vi "Database.UpdateVariantFiles.vi"(8 "error in":errorcluster) -> (0 "error out":errorcluster)   [LabVIEW 2016]
uses:
  Global/ApplicationGlobal.vi
  Logger/Logger.FileBody.ctl
panel:
  out "HandledFileContent":T1[](array[typedef]) {"Values" format="%.3f"}
  out "HandledFileContent":T1 {"Values" format="%.3f"}
  out "Array":string[](array[string])
  out "text":string
  out "SerialNo":string
  out "Variant":string
  out "System":string
  out "filenames":string[](array[string])
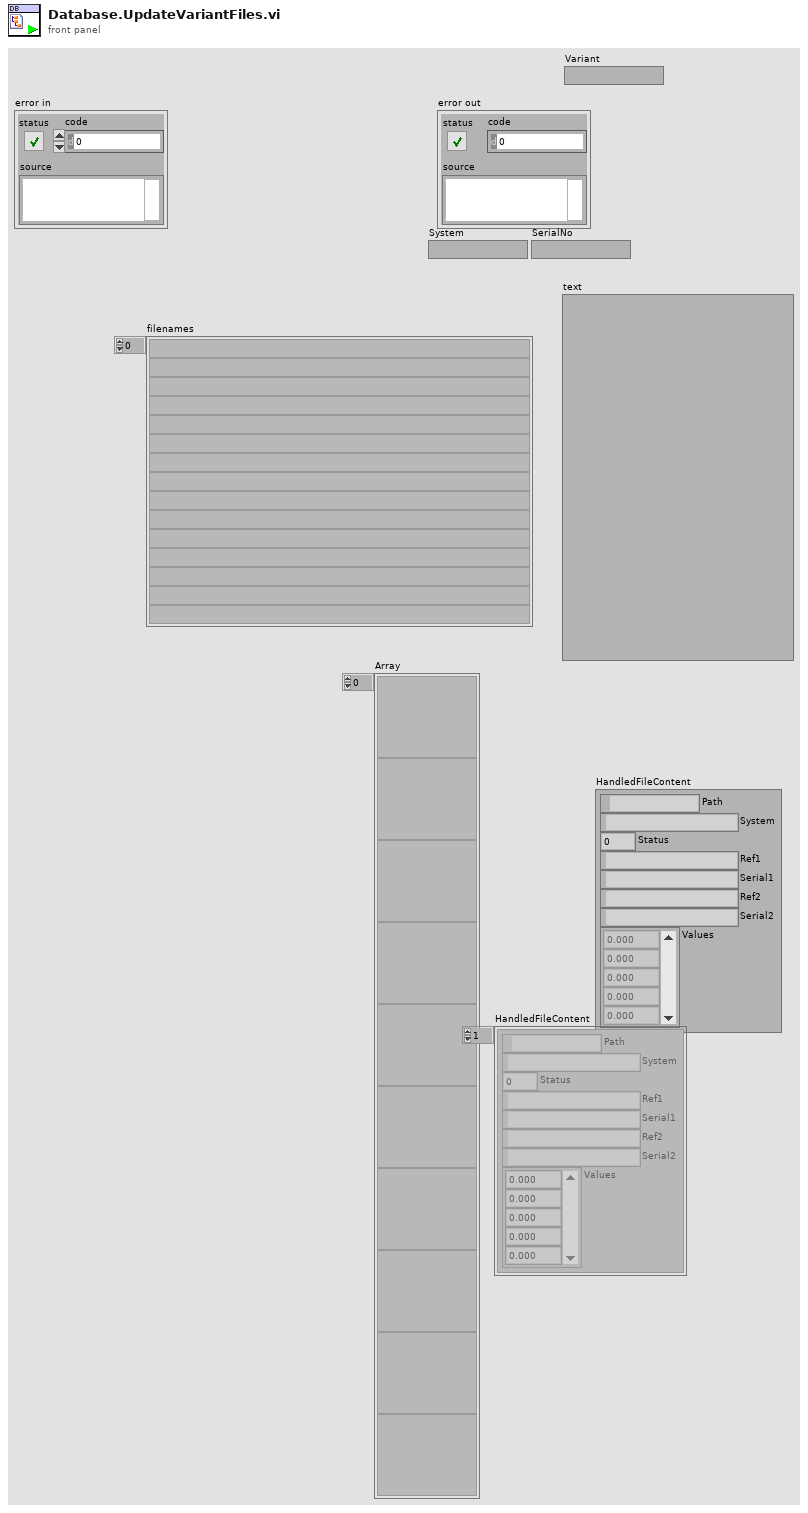
[diagram p1: front panel]
types:
  T1 = typedef "Logger.FileBody.ctl" = cluster{"Path":path, "System":string, "Status":u8, "Ref1":string, "Serial1":string, "Ref2":string, "Serial2":string, "Values":sgl[]}
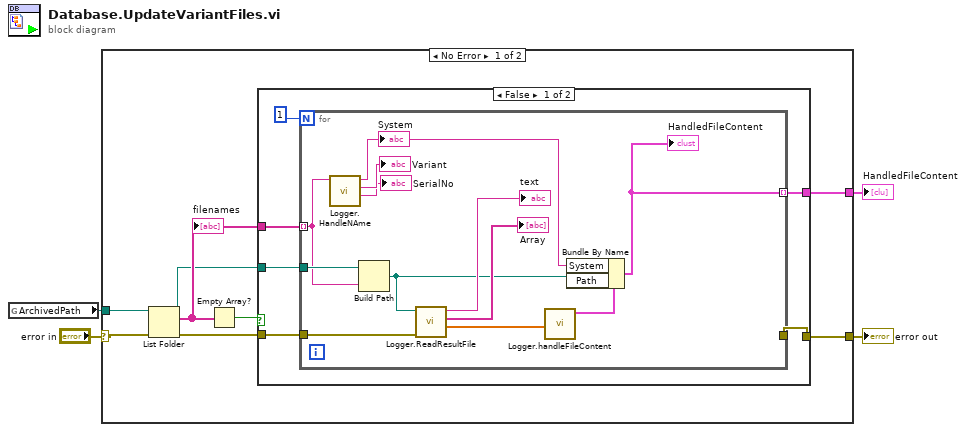
[diagram p0: block diagram]
diagram:
  n1 = global read "ApplicationGlobal.vi" "ArchivedPath"() -> (w2:path)
  n2 = case shown="No Error" "error in" {
    selector: "error in" -> [w11 w34]
    tunnel: [w5 w34] -> w4
    tunnel: w2 -> [w12 _]
    tunnel: [w7 _] -> w1
    frame No Error {
      n3 = List Folder(path=w12, error in=w11) -> (path out=w8:path, filenames=w9:string[], error out=w6:errorcluster)  [unwired: 2 in, 1 out]
      "filenames" <- w9
      n4 = Empty Array?(array=w9) -> (empty?=w10:bool)
      n5 = case shown="False" w10 {
        tunnel: w9 -> [w18 _]
        tunnel: w8 -> [w17 _]
        tunnel: [w16 _] -> w7
        tunnel: w6 -> [w15 w33]
        tunnel: [w14 w33] -> w5
        frame False {
          n6 = for {
            N: 1 -> [_]
            tunnel: w18 -> [w29] mode=indexing
            tunnel: w17 -> [w30]
            tunnel: [w21] -> w16 mode=indexing
            tunnel: w15 -> [w25]
            tunnel: [w20] -> w14
            n7 = call "Logger.HandleNAme.vi"("String"=w29) -> ("SerialNo"=→"SerialNo":string, "Variant"=→"Variant":string, "System"=w23:string)  [unwired: 8 in]
            "System" <- w23
            n8 = Build Path(base path=w30, name or relative path=w29) -> (appended path=w24:path)
            n9 = call "Logger.ReadResultFile.vi"("error in"=w25, "ResultFilePath"=w24) -> ("error out"=w22:errorcluster, 1:"ResultValues"=w28:dbl[], 2:"ResultValues"=→"Array":string[], "text"=→"text":string)  [unwired: 6 in]
            n10 = call "Logger.handleFileContent.vi"("ResultsFile"=w28) -> ("HandledFileContent"=w19:T1)  [unwired: 10 in]
            n11 = Bundle By Name(cluster=w19, "System"=w23, "Path"=w24) -> (w21:T1)
            "HandledFileContent" <- w21
          }
        }
        frame True {
        }
      }
    }
    frame Error {
    }
  }
  "error out" <- w4
  "HandledFileContent" <- w1
